vi "Read Name core.vi"(11 "Build Item in":refnum<class "Create ZIP Step.lvclass">) -> (2 "Name":string)   [LabVIEW 2019, in "ZIP.lvlib" / "Create ZIP Step.lvclass"]
doc: "Gets the name for the build step\n\nCopyright: MGI 2016\nAuthor: Derek Trepanier"
uses:
  Create ZIP Step.lvclass
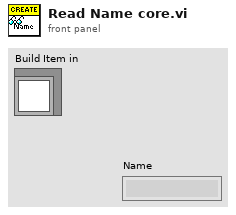
[diagram p1: front panel]
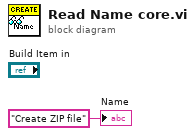
[diagram p0: block diagram]
diagram:
  "Name" <- "Create ZIP file" ("Name")
